vi "Destructor.vi"(8 "error in (no error)":errorcluster, 11 "Aalborg GFC17 in":refnum<class "Aalborg GFC17.lvclass">) -> (0 "error out":errorcluster, 3 "Aalborg GFC17 out":refnum<class "Aalborg GFC17.lvclass">)   [LabVIEW 2011, in "Aalborg GFC17.lvclass"]
uses:
  Aalborg GFC17.lvclass
  Mass Flow Controller/Valve Status.ctl
  Aalborg GFC17.lvclass/Aalborg GFC17.ctl
  Mass Flow Controller/Mass Flow Controller.lvclass
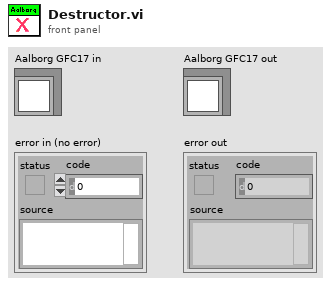
[diagram p1: front panel]
types:
  T1 = typedef "Mass Flow Controller.lvclass/Valve Status.ctl" = enum16{"Open", "Closed"}
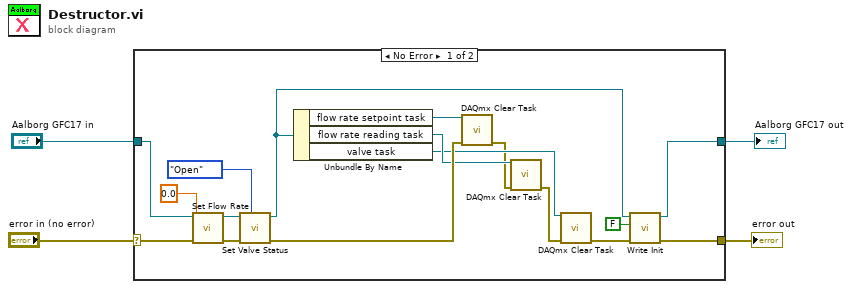
[diagram p0: block diagram]
diagram:
  n1 = case shown="No Error" "error in (no error)" {
    selector: "error in (no error)" -> [w16 w23]
    tunnel: [w11 w23] -> w3
    tunnel: [w12 w22] -> w1
    tunnel: "Aalborg GFC17 in" -> [w15 w22]
    frame No Error {
      n2 = call-dynamic "Set Flow Rate.vi"("error in (no error)"=w16, "Flow Rate"=0.0, "Aalborg GFC17 in"=w15) -> ("error out"=w20:errorcluster, "Aalborg GFC17 out"=w19:refnum<class "Aalborg GFC17.lvclass">)  [unwired: 7 in]
      n3 = call-dynamic "Set Valve Status.vi"("Valve Status"=Valve_Status."Open", "error in (no error)"=w20, "Aalborg GFC17 in"=w19) -> ("error out"=w9:errorcluster, "Aalborg GFC17 out"=w5:refnum<class "Aalborg GFC17.lvclass">)  [unwired: 7 in]
      n4 = Unbundle By Name(w5) -> ("flow rate setpoint task"=w10:refnum<k21>, "flow rate reading task"=w8:refnum<k21>, "valve task"=w7:refnum<k21>)
      n5 = call <vilib>:"DAQmx Clear Task.vi"("task in"=w10, "error in"=w9) -> ("error out"=w6:errorcluster)  [unwired: 13 in]
      n6 = call <vilib>:"DAQmx Clear Task.vi"("task in"=w8, "error in"=w6) -> ("error out"=w21:errorcluster)  [unwired: 13 in]
      n7 = call <vilib>:"DAQmx Clear Task.vi"("task in"=w7, "error in"=w21) -> ("error out"=w14:errorcluster)  [unwired: 13 in]
      n8 = call-dynamic "Write Init.vi"("error in (no error)"=w14, "Init"=FALSE, "Mass Flow Controller in"=w5) -> ("error out"=w11:errorcluster, "Mass Flow Controller out"=w12:refnum<class "Aalborg GFC17.lvclass">)  [unwired: 7 in]
    }
    frame Error {
    }
  }
  "error out" <- w3
  "Aalborg GFC17 out" <- w1
